vi "Get Task for Task Kind.vi"(9 "DAQmx Task prefix":string, 11 "Task Map in":map{string, refnum<k21>}(c390)) -> (1 "DAQmx Task":refnum<k21>, 2 "key not found?":bool, 3 "Task Map out":map{string, refnum<k21>}(c390))   [LabVIEW 2021, in "Load Frame.lvlib"]
doc: "Get the Task that matches the 'DAQmx Task prefix' from the Task Map."
uses:
  Load Frame.lvlib
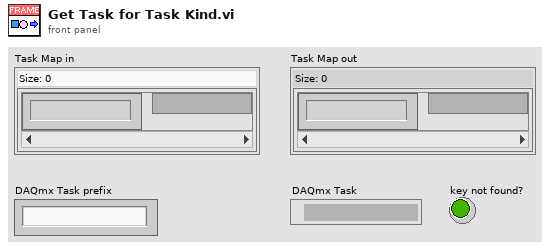
[diagram p1: front panel]
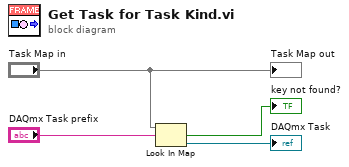
[diagram p0: block diagram]
diagram:
  n1 = Look In Map(map="Task Map in", key="DAQmx Task prefix") -> (key not found?=→"key not found?":bool, value=→"DAQmx Task":refnum<k21>)  [unwired: 1 in]
  "Task Map out" <- "Task Map in"
